vi "Write_Indexes.vi"(2 "analogue Indexes":T1, 3 "digital Indexes":cluster{"Start index":u16, "Stop index":u16}, 4 "indexesAddress":u32) -> (0 "Error Out":u8, 1 "Aborted":bool)   [LabVIEW 2017]
uses:
  <vilib>/rvi/Memory/Memory_Emulation/nirvimemoryFastEmulation.vi
  <vilib>/rvi/Memory/Memory_Emulation/nirvimemoryEmulation.vi
  <vilib>/rvi/Emulation/niFpgaEmulationIsFPGAContextNoSignature.vi
  <vilib>/rvi/DataTransferAndStorage/Container/Common/niFpgaContainerGetUniqueNameForEmu.vi
  <vilib>/rvi/Emulation/niFpgaProcessEmulError.vi
  <vilib>/rvi/Emulation/niFpgaSctlEmulationGetInTimedLoop.vi
  <vilib>/rvi/errors/nirviReportUnexpectedCaseInternalError (U32).vi
  <vilib>/rvi/DataTransferAndStorage/Container/XNode/niFpgaContainer.xnode
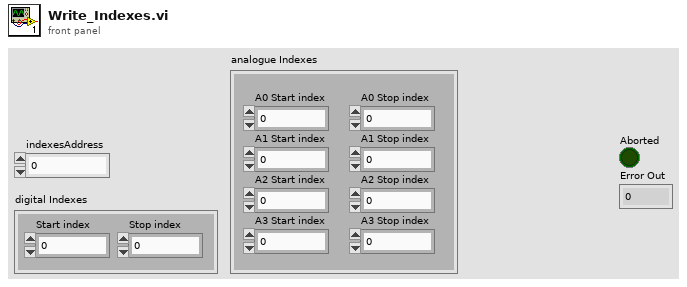
[diagram p1: front panel]
types:
  T1 = cluster{"A0 Start index":u16, "A0 Stop index":u16, "A1 Start index":u16, "A1 Stop index":u16, "A2 Start index":u16, "A2 Stop index":u16, "A3 Start index":u16, "A3 Stop index":u16}
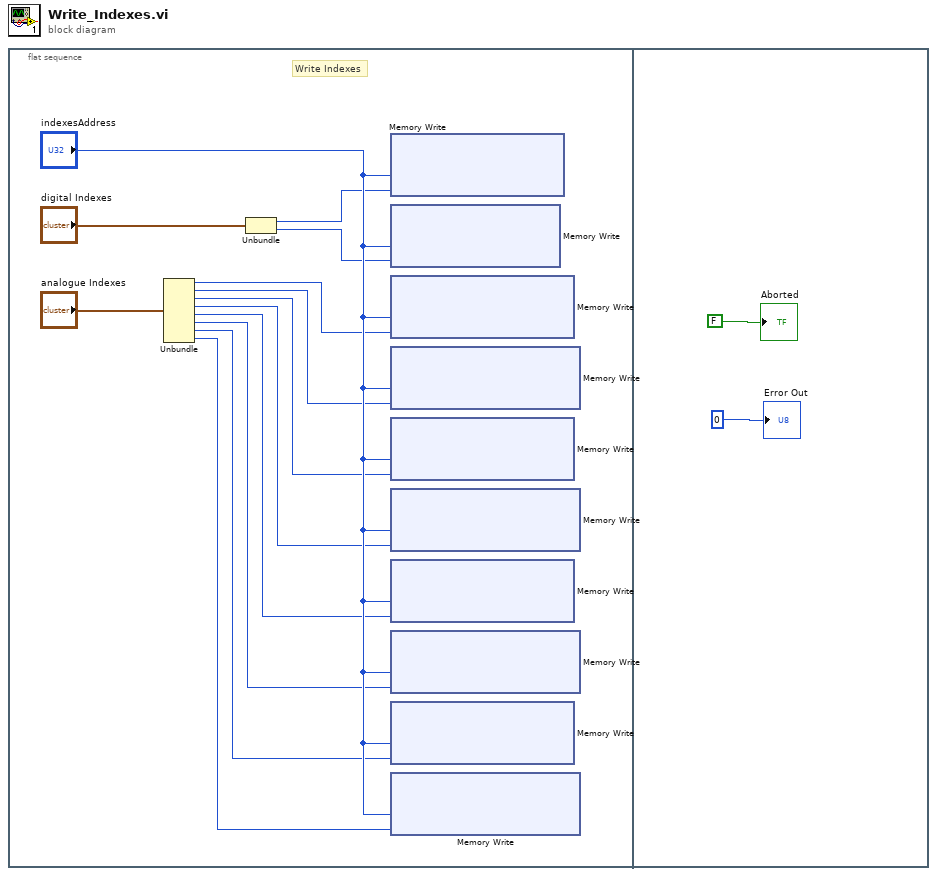
[diagram p0: block diagram]
diagram:
  n1 = flat-sequence {
    frame #0 {
      # "Write Indexes"
      n2 = Unbundle("analogue Indexes") -> ("A0 Start index"=w3:u16, "A0 Stop index"=w4:u16, "A1 Start index"=w5:u16, "A1 Stop index"=w6:u16, "A2 Start index"=w7:u16, "A2 Stop index"=w8:u16, "A3 Start index"=w9:u16, "A3 Stop index"=w10:u16)
      n3 = Unbundle("digital Indexes") -> ("Start index"=w1:u16, "Stop index"=w2:u16)
      n4 = xnode ("Memory Write")("Address"="indexesAddress", "Data"=w1) -> ()  [unwired: 1 in, 1 out]
      n5 = xnode ("Memory Write")("Address"="indexesAddress", "Data"=w2) -> ()  [unwired: 1 in, 1 out]
      n6 = xnode ("Memory Write")("Address"="indexesAddress", "Data"=w3) -> ()  [unwired: 1 in, 1 out]
      n7 = xnode ("Memory Write")("Address"="indexesAddress", "Data"=w4) -> ()  [unwired: 1 in, 1 out]
      n8 = xnode ("Memory Write")("Address"="indexesAddress", "Data"=w5) -> ()  [unwired: 1 in, 1 out]
      n9 = xnode ("Memory Write")("Address"="indexesAddress", "Data"=w6) -> ()  [unwired: 1 in, 1 out]
      n10 = xnode ("Memory Write")("Address"="indexesAddress", "Data"=w7) -> ()  [unwired: 1 in, 1 out]
      n11 = xnode ("Memory Write")("Address"="indexesAddress", "Data"=w8) -> ()  [unwired: 1 in, 1 out]
      n12 = xnode ("Memory Write")("Address"="indexesAddress", "Data"=w9) -> ()  [unwired: 1 in, 1 out]
      n13 = xnode ("Memory Write")("Address"="indexesAddress", "Data"=w10) -> ()  [unwired: 1 in, 1 out]
    }
    frame #1 {
      "Aborted" <- FALSE
      "Error Out" <- u8 0
    }
  }
